vi "GetUIRef.vi"(8 "error in (no error)":errorcluster, 11 "MGI_Progress Bar in":refnum<class "Progress Bar.lvclass">) -> (0 "error out":errorcluster, 2 "VI Refnum":refnum<vi>, 3 "MGI_Progress Bar out":refnum<class "Progress Bar.lvclass">)   [LabVIEW 2020, in "Progress Bar.lvclass"]
doc: "Gets a reference to the UI VI. If you're interested in customizing the look of the progress bar, you'll need to overide this function to make sure it points to your new UI VI\n\nCopyright: MGI\nAuthored by: Derek Trepanier"
uses:
  <userlib>/_MGI/User Interface/Progress Bar/Progress Bar.lvclass
  <userlib>/_MGI/User Interface/Progress Bar/Progress Bar Settings/Progress Bar Settings.lvclass
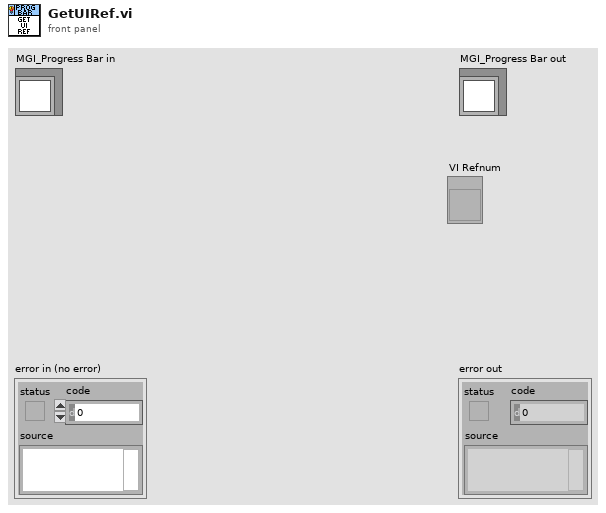
[diagram p1: front panel]
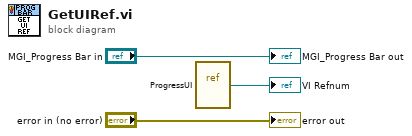
[diagram p0: block diagram]
diagram:
  n1 = vi-ref <userlib>:"ProgressUI.vi"() -> (→"VI Refnum":refnum<vi>)
  "error out" <- "error in (no error)"
  "MGI_Progress Bar out" <- "MGI_Progress Bar in"
